vi "getXMLHeader.vi"() -> (2 "xml header":string)   [LabVIEW 2009, in "Caraya.lvlib" / "Test Report.JUnit.lvclass"]
uses:
  Test Report.JUnit.lvclass
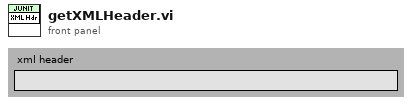
[diagram p1: front panel]
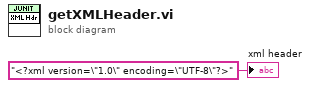
[diagram p0: block diagram]
diagram:
  "xml header" <- "<?xml version=\"1.0\" encoding=\"UTF-8\"?>" ("xml header")
